vi "main.vi"(8 "error in (no error)":errorcluster) -> (0 "error out":errorcluster)   [LabVIEW 2015, in "lv-interface-nre.lvlib"]
uses:
  lv-interface-nre.lvlib
  private/_controls/hmi_references.ctl
  private/_controls/hmi_states.ctl
  private/_controls/event_common.ctl
  private/_controls/event_common_command.ctl
  private/_controls/event_interface.ctl
  private/_controls/event_interface_command.ctl
  private/_controls/menu_selection.ctl
panel:
  out "time_date":dbl format="%<%H:%M:%S%3u\n%m/%d/%y>T"
  in  "refresh_rate_ms":i32=1000
  out "random_number":dbl
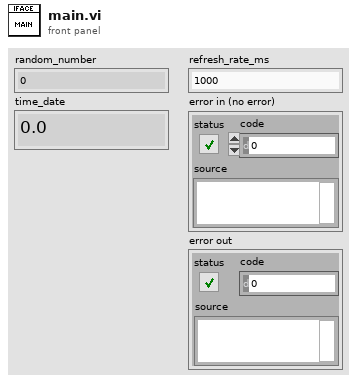
[diagram p1: front panel]
types:
  T1 = typedef "lv-interface-nre.lvlib/hmi_references.ctl" = cluster{"vi_reference":refnum<vi>}
  T2 = typedef "lv-interface-nre.lvlib/event_interface.ctl" = cluster{"command":T3, "data":variant}
  T3 = typedef "lv-interface-nre.lvlib/event_interface_command.ctl" = enum16{"<event_interface_cmd>", "defer_panel_updates", "undefer_panel_updates", "<null>"}
  T4 = typedef "lv-interface-nre.lvlib/event_common.ctl" = cluster{"command":T5, "data":variant}
  T5 = typedef "lv-interface-nre.lvlib/event_common_command.ctl" = enum16{"<event_common_cmd>", "die", "<null>"}
  T6 = typedef "lv-interface-nre.lvlib/hmi_states.ctl" = enum16{"<hmi_states>", "initialize", "checkui", "shutdown", "<null>"}
  T7 = typedef "lv-interface-nre.lvlib/menu_selection.ctl" = enum16{"<menu>", "file_exit", "help_about", "<null>"}
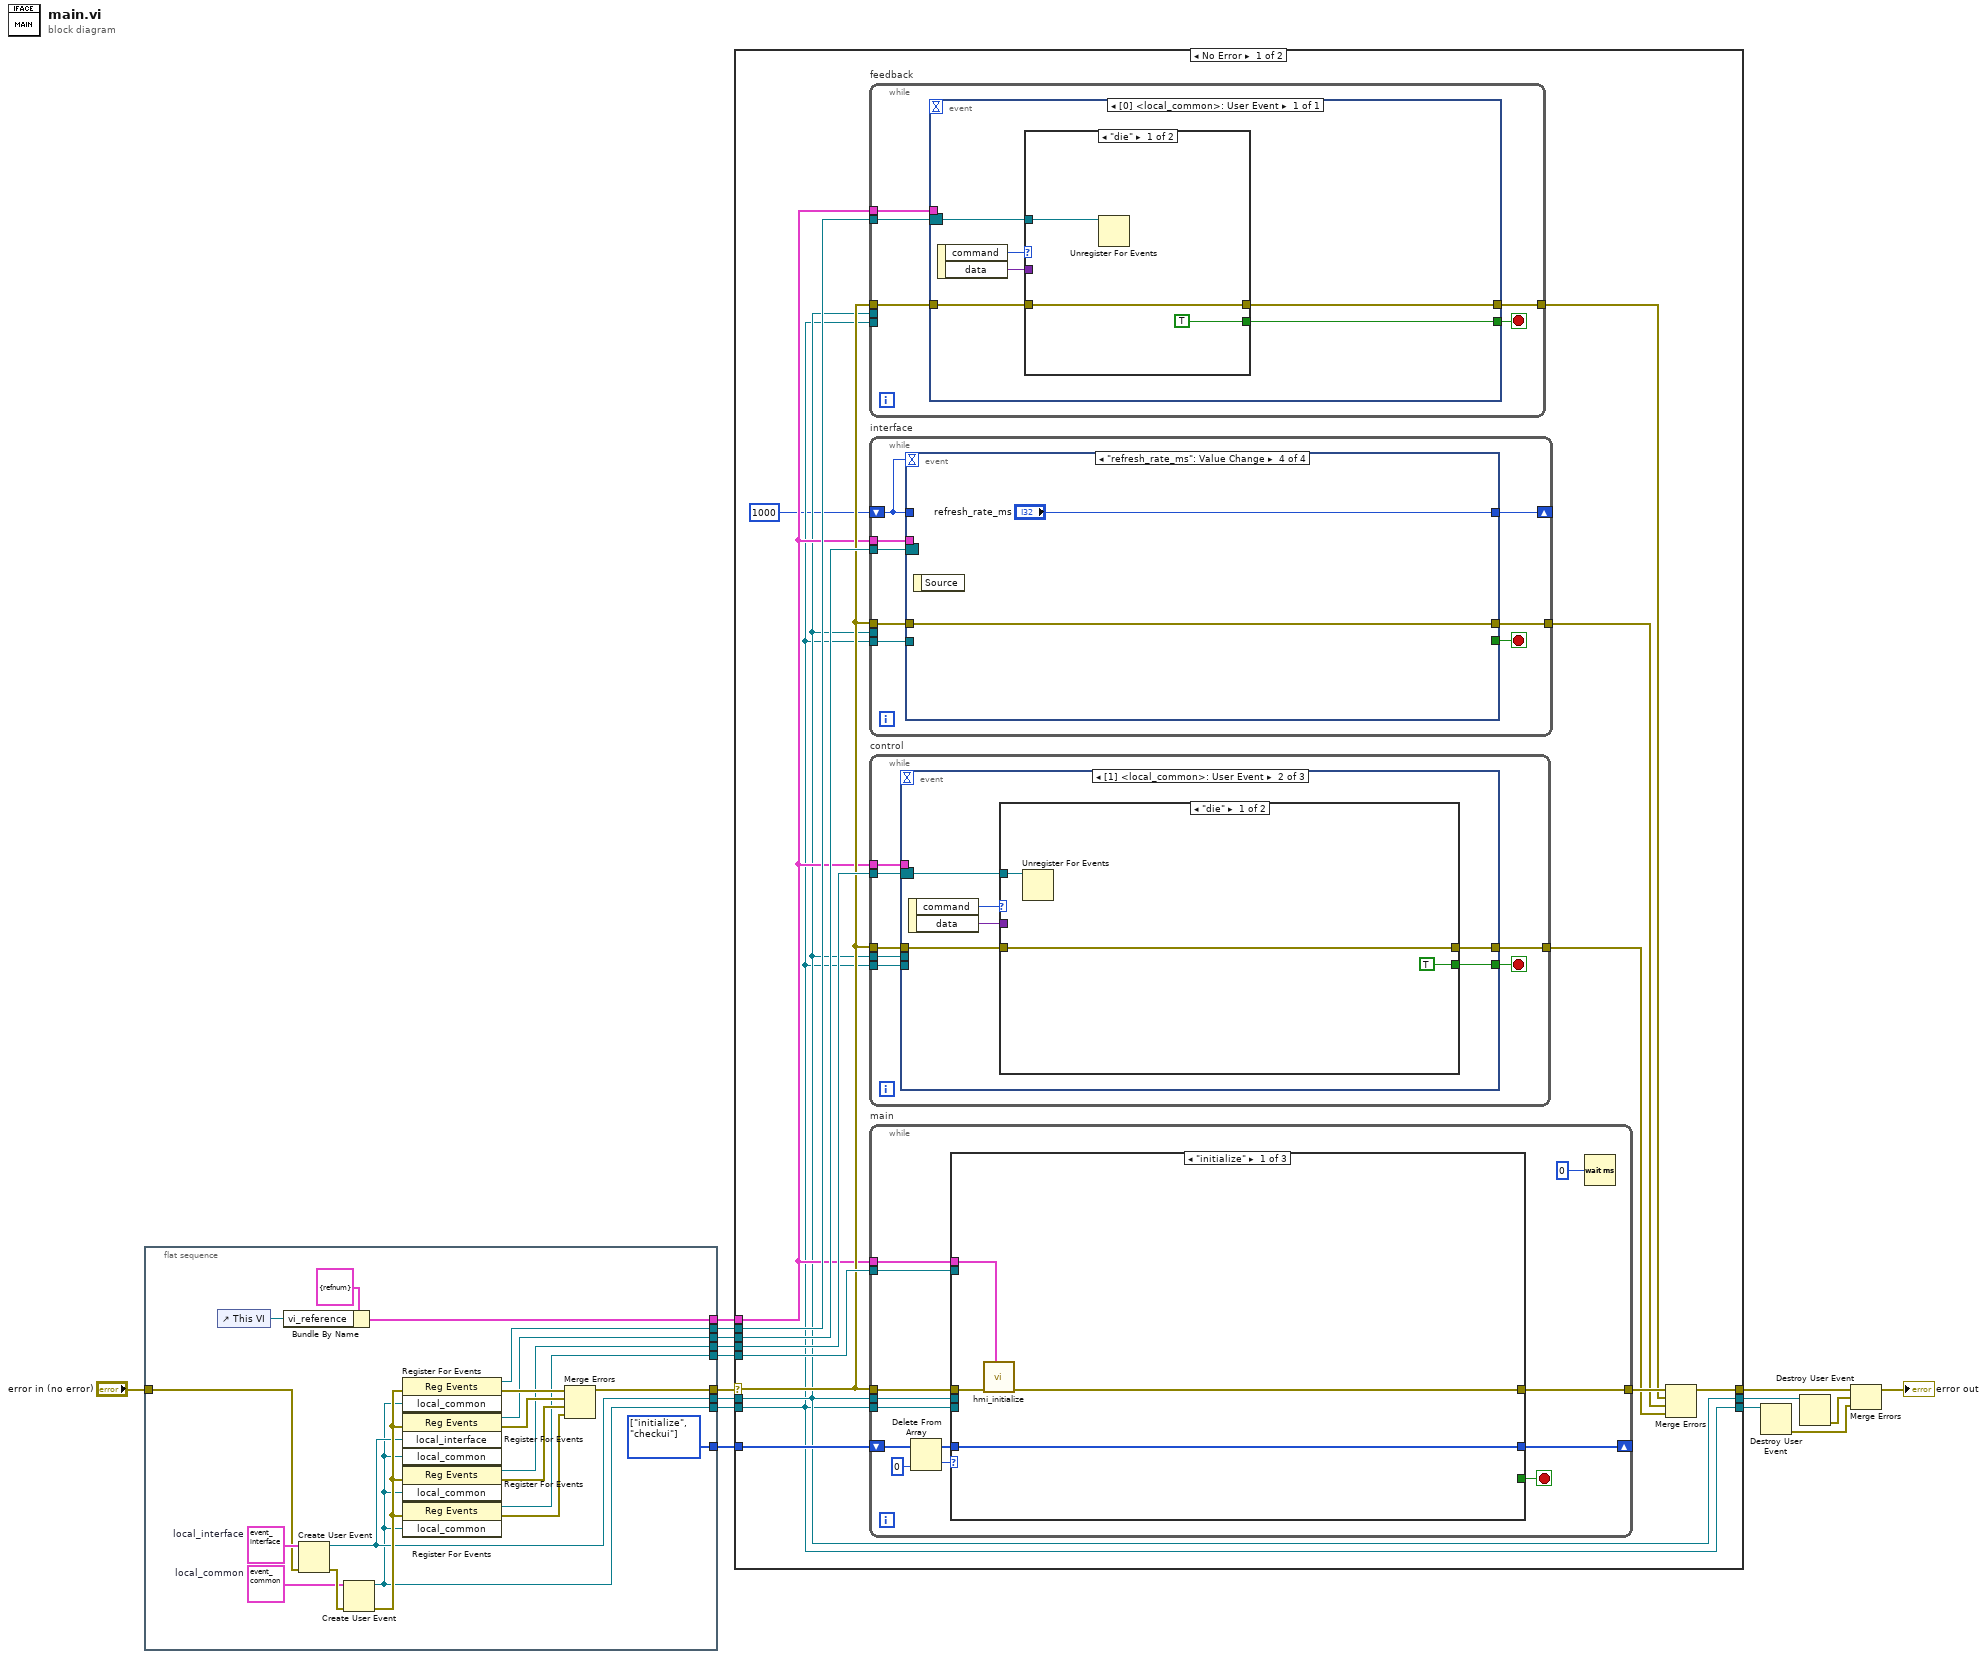
[diagram p0: block diagram]
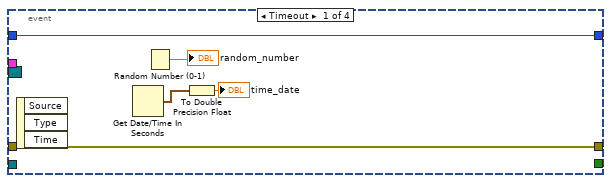
[diagram p3: hidden frame]
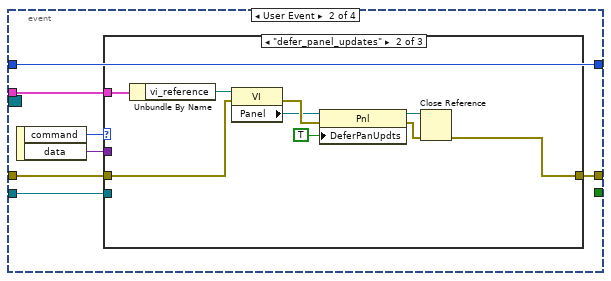
[diagram p4: hidden frame]
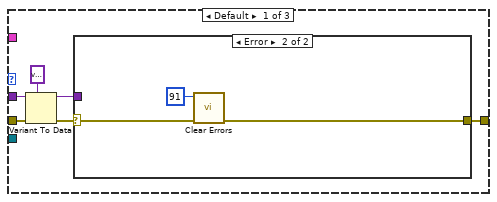
[diagram p5: hidden frame]
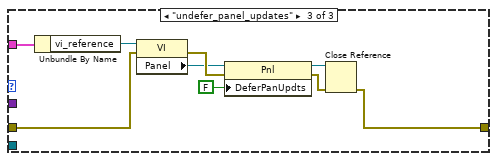
[diagram p7: hidden frame]
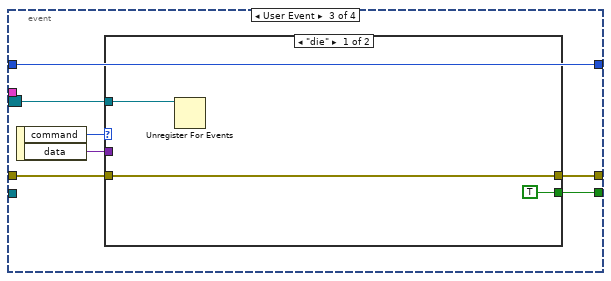
[diagram p8: hidden frame]
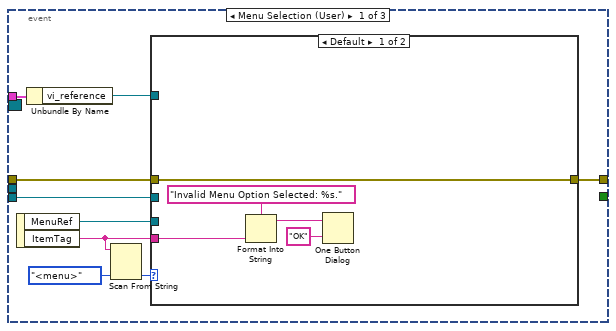
[diagram p10: hidden frame]
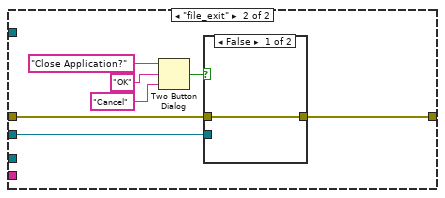
[diagram p11: hidden frame]
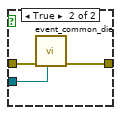
[diagram p12: hidden frame]
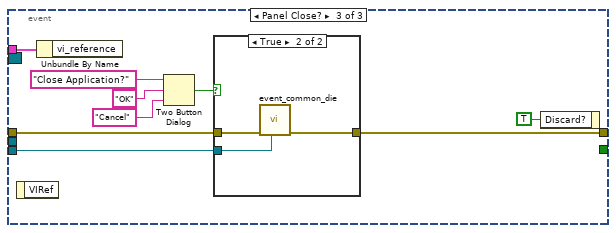
[diagram p14: hidden frame]
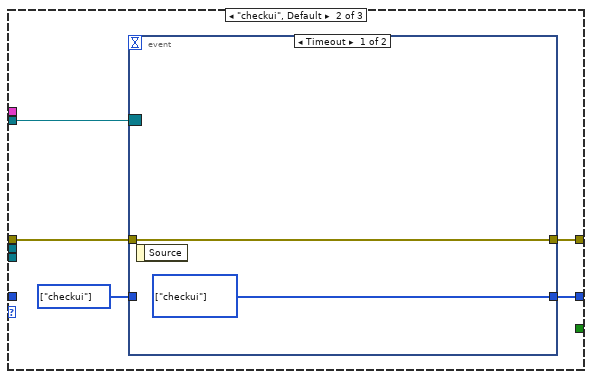
[diagram p16: hidden frame]
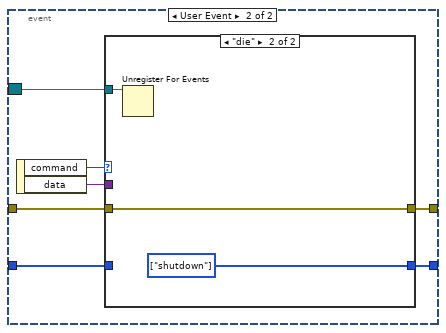
[diagram p17: hidden frame]
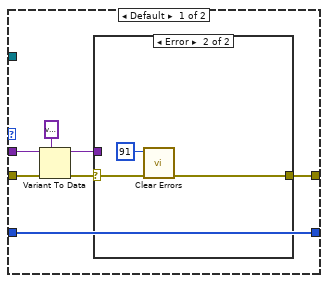
[diagram p18: hidden frame]
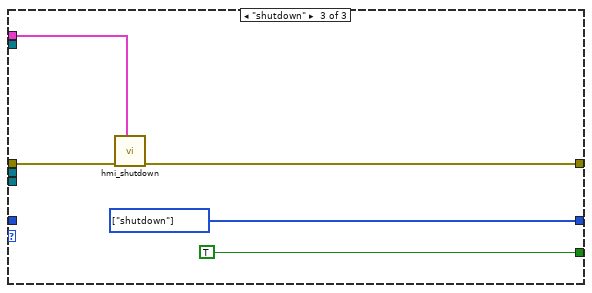
[diagram p20: hidden frame]
diagram:
  n1 = flat-sequence {
    tunnel: [w28] -> w16
    tunnel: [w27] -> w15
    tunnel: [w31] -> w14
    tunnel: "error in (no error)" -> [w17]
    tunnel: [w26] -> w12
    tunnel: [w25] -> w11
    tunnel: [w23] -> w10
    tunnel: [w19] -> w8
    tunnel: [w20] -> w9
    tunnel: [w18] -> w2
    frame #0 {
      w21 = T2 {"command"=enum."<event_interface_cmd>", "data"=variant}  # local_interface
      w22 = T4 {"command"=enum."<event_common_cmd>", "data"=variant}  # local_common
      w31 = T6[] [enum."initialize", enum."checkui"] items=["<hmi_states>", "initialize", "checkui", "shutdown", "<null>"]
      n2 = control-ref of="This VI"() -> (w24:refnum<vi>)
      n3 = Bundle By Name(cluster=T1 {"vi_reference"=refnum}, "vi_reference"=w24) -> (w23:T1)
      n4 = Create User Event(user event datatype=w21, error in=w17) -> (user event=w20:refnum<user-event>, error out=w35:errorcluster)
      n5 = Create User Event(user event datatype=w22, error in=w35) -> (user event=w19:refnum<user-event>, error out=w34:errorcluster)
      n6 = register-events(error in=w34, w19) -> (reference out=w18:refnum<event-registration>, error out=w36:errorcluster)  [unwired: 1 in]
      n7 = register-events(error in=w34, w20, w19) -> (reference out=w25:refnum<event-registration>, error out=w33:errorcluster)  [unwired: 1 in]
      n8 = register-events(error in=w34, w19) -> (reference out=w27:refnum<event-registration>, error out=w30:errorcluster)  [unwired: 1 in]
      n9 = register-events(error in=w34, w19) -> (reference out=w26:refnum<event-registration>, error out=w29:errorcluster)  [unwired: 1 in]
      n10 = Merge Errors(w36, w33, w30, w29) -> (w28:errorcluster)
    }
  }
  n11 = case shown="No Error" w16 {
    selector: w16 -> [w42 w239]
    tunnel: w15 -> [w45 w235]
    tunnel: w14 -> [w47 _]
    tunnel: [w43 w239] -> w5
    tunnel: w12 -> [w46 w234]
    tunnel: w11 -> [w44 w236]
    tunnel: w10 -> [w41 _]
    tunnel: w9 -> [w40 w238]
    tunnel: w8 -> [w39 w237]
    tunnel: [w40 w238] -> w6
    tunnel: [w39 w237] -> w7
    tunnel: w2 -> [w51 w233]
    frame No Error {
      n12 = while "feedback" {
        tunnel: [w56] -> w38
        tunnel: w42 -> [w55]
        tunnel: w51 -> [w54]
        tunnel: w41 -> [w53]
        tunnel: w40 -> [_]
        tunnel: w39 -> [_]
        stop <- w52 stop-if-true
        n13 = event shown="[0] <local_common>: User Event" {
          selector: w54 -> [w62]
          dyn-events: _ -> [_]
          timeout: _ -> [_]
          tunnel: [w59] -> w56
          tunnel: w55 -> [w60]
          tunnel: w53 -> [_]
          tunnel: [w58] -> w52
          event User Event {
            n14 = event-data() -> ("command"=w61:T5, "data"=w57:variant)  [unwired: 1 in]
            n15 = case shown="\"die\"" w61 {
              tunnel: w60 -> [w64 w66]
              tunnel: [w64 w66] -> w59
              tunnel: [TRUE _] -> w58
              tunnel: w62 -> [w63 _]
              tunnel: w57 -> [_ _]
              frame "die" {
                n16 = Unregister For Events(event registration refnum=w63) -> ()  [unwired: 1 in, 1 out]
              }
              frame Default {
              }
            }
          }
        }
      }
      n17 = while "interface" {
        tunnel: w42 -> [w74]
        tunnel: [w72] -> w48
        tunnel: w44 -> [w71]
        tunnel: w40 -> [_]
        tunnel: w39 -> [w70]
        tunnel: w41 -> [w69]
        shift-right: [w67] -> _
        shift-left: 1000 ("refresh_rate_ms") -> [w68]
        stop <- w73 stop-if-true
        n18 = event shown="[3] \"refresh_rate_ms\": Value Change" {
          selector: w71 -> [_ _ w117 _]
          dyn-events: _ -> [_ _ _ _]
          timeout: w68 -> [_ _ _ _]
          tunnel: w74 -> [w77 w84 w120 w126]
          tunnel: [w77 w83 w119 w126] -> w72
          tunnel: [_ _ w118 _] -> w73
          tunnel: w70 -> [_ w82 _ _]
          tunnel: w69 -> [_ w81 _ _]
          tunnel: w68 -> [w79 w80 w115 _]
          tunnel: [w79 w80 w115 "refresh_rate_ms"] -> w67
          event Timeout {
            n19 = event-data() -> ()  [unwired: 1 in, 3 out]
            n20 = Get Date/Time In Seconds() -> (seconds since 1Jan1904=w76:timestamp)
            n21 = Random Number (0-1)() -> (number: 0 to 1=→"random_number":dbl)
            n22 = To Double Precision Float(number=w76) -> (double precision float=→"time_date":dbl)
          }
          event User Event {
            n23 = event-data() -> ("command"=w86:T3, "data"=w85:variant)  [unwired: 1 in]
            n24 = case shown="\"defer_panel_updates\"" w86 {
              tunnel: w84 -> [w91 w100 w109]
              tunnel: [w87 w99 w106] -> w83
              tunnel: w85 -> [w92 _ _]
              tunnel: w82 -> [_ _ _]
              tunnel: w81 -> [_ w98 w108]
              frame Default {
                n25 = Variant To Data(error in=w91, type=variant, Variant=w92) -> (data=w88:variant, error out=w90:errorcluster)
                n26 = case shown="Error" w90 {
                  selector: w90 -> [w93 w96]
                  tunnel: w88 -> [_ _]
                  tunnel: [w93 w95] -> w87
                  frame No Error {
                  }
                  frame Error {
                    n27 = call <vilib>:"Clear Errors.vi"("error in (no error)"=w96, "specific error code to clear (0: all)"=91) -> ("error out"=w95:errorcluster)  [unwired: 4 in, 1 out]
                  }
                }
              }
              frame "defer_panel_updates" {
                n28 = Unbundle By Name(w98) -> ("vi_reference"=w97:refnum<vi>)
                n29 = property class="VI"(reference=w97, error in=w100) -> (error out=w105:errorcluster, "Panel"=w101:refnum<vi>)  [unwired: 1 out]
                n30 = property class="Pnl"(reference=w101, error in=w105, "DeferPanUpdts"=TRUE ("Defer Panel Updates")) -> (reference out=w103:refnum<vi>, error out=w102:errorcluster)
                n31 = Close Reference(reference=w103, error in (no error)=w102) -> (error out=w99:errorcluster)
              }
              frame "undefer_panel_updates" {
                n32 = Unbundle By Name(w108) -> ("vi_reference"=w107:refnum<vi>)
                n33 = property class="VI"(reference=w107, error in=w109) -> (error out=w114:errorcluster, "Panel"=w110:refnum<vi>)  [unwired: 1 out]
                n34 = property class="Pnl"(reference=w110, error in=w114, "DeferPanUpdts"=FALSE ("Defer Panel Updates")) -> (reference out=w112:refnum<vi>, error out=w111:errorcluster)
                n35 = Close Reference(reference=w112, error in (no error)=w111) -> (error out=w106:errorcluster)
              }
            }
          }
          event User Event {
            n36 = event-data() -> ("command"=w121:T5, "data"=w116:variant)  [unwired: 1 in]
            n37 = case shown="\"die\"" w121 {
              tunnel: w120 -> [w123 w125]
              tunnel: [w123 w125] -> w119
              tunnel: [TRUE _] -> w118
              tunnel: w117 -> [w122 _]
              tunnel: w116 -> [_ _]
              frame "die" {
                n38 = Unregister For Events(event registration refnum=w122) -> ()  [unwired: 1 in, 1 out]
              }
              frame Default {
              }
            }
          }
          event "refresh_rate_ms": Value Change {
            n39 = event-data() -> ()  [unwired: 1 in, 1 out]
          }
        }
      }
      n40 = while "control" {
        tunnel: w42 -> [w134]
        tunnel: [w132] -> w49
        tunnel: w45 -> [w131]
        tunnel: w40 -> [w129]
        tunnel: w39 -> [w128]
        tunnel: w41 -> [w130]
        stop <- w133 stop-if-true
        n41 = event shown="[1] <local_common>: User Event" {
          selector: w131 -> [_ w160 _]
          dyn-events: _ -> [_ _ _]
          timeout: _ -> [_ _ _]
          tunnel: w134 -> [w140 w164 w170]
          tunnel: [w138 w163 w177] -> w132
          tunnel: [_ w162 _] -> w133
          tunnel: w130 -> [w137 _ w176]
          tunnel: w129 -> [_ _ _]
          tunnel: w128 -> [w135 _ w175]
          event Menu Selection (User) {
            n42 = event-data() -> ("MenuRef"=w141:refnum<k9>, "ItemTag"=w139:string)  [unwired: 1 in]
            n43 = Unbundle By Name(w137) -> ("vi_reference"=w136:refnum<vi>)
            n44 = Scan From String(input string=w139, default 1=menu_selection."<menu>" ("menu_selection")) -> (output 1=w142:T7)  [unwired: 3 in, 3 out]
            n45 = case shown="Default" w142 {
              tunnel: w141 -> [_ _]
              tunnel: w140 -> [w144 w149]
              tunnel: w139 -> [w148 _]
              tunnel: [w144 w155] -> w138
              tunnel: w136 -> [_ _]
              tunnel: w135 -> [_ w154]
              frame Default {
                n46 = Format Into String(format string="Invalid Menu Option Selected: %s.", w148) -> (resulting string=w146:string)  [unwired: 2 in, 1 out]
                n47 = One Button Dialog(message=w146, button name ("OK")="OK" ("boolean_text_1")) -> ()  [unwired: 1 out]
              }
              frame "file_exit" {
                n48 = Two Button Dialog(message="Close Application?" ("dialog_text"), 1:"Cancel" ("boolean_text_1"), 2:"OK" ("boolean_text_1")) -> (T button?=w150:bool)
                n49 = case shown="False" w150 {
                  tunnel: w149 -> [w156 w159]
                  tunnel: [w156 w158] -> w155
                  tunnel: w154 -> [_ w157]
                  frame False {
                  }
                  frame True {
                    n50 = call "event_common_die.vi"("local_common"=w157, "error in (no error)"=w159) -> ("error out"=w158:errorcluster)  [unwired: 9 in]
                  }
                }
              }
            }
          }
          event User Event {
            n51 = event-data() -> ("command"=w165:T5, "data"=w161:variant)  [unwired: 1 in]
            n52 = case shown="\"die\"" w165 {
              tunnel: w164 -> [w166 w169]
              tunnel: [w166 w169] -> w163
              tunnel: [TRUE _] -> w162
              tunnel: w161 -> [_ _]
              tunnel: w160 -> [w167 _]
              frame "die" {
                n53 = Unregister For Events(event registration refnum=w167) -> ()  [unwired: 1 in, 1 out]
              }
              frame Default {
              }
            }
          }
          event Panel Close? {
            n54 = event-data() -> ()  [unwired: 1 in, 1 out]
            n55 = Unbundle By Name(w176) -> ()  [unwired: 1 out]
            n56 = Two Button Dialog(message="Close Application?" ("dialog_text"), 1:"Cancel" ("boolean_text_1"), 2:"OK" ("boolean_text_1")) -> (T button?=w171:bool)
            n57 = case shown="True" w171 {
              tunnel: w170 -> [w179 w182]
              tunnel: [w179 w181] -> w177
              tunnel: w175 -> [_ w180]
              frame False {
              }
              frame True {
                n58 = call "event_common_die.vi"("local_common"=w180, "error in (no error)"=w182) -> ("error out"=w181:errorcluster)  [unwired: 9 in]
              }
            }
            n59 = event-data("Discard?"=TRUE) -> ()  [unwired: 1 in, 1 out]
          }
        }
      }
      n60 = while "main" {
        shift-right: [w187] -> _
        shift-left: w47 -> [w194]
        tunnel: w46 -> [w188]
        tunnel: w42 -> [w190]
        tunnel: [w186] -> w50
        tunnel: w41 -> [w185]
        tunnel: w39 -> [w184]
        tunnel: w40 -> [w183]
        stop <- w189 stop-if-true
        n61 = Delete From Array(array=w194, index=0) -> (deleted portion=w192:T6, array with subset deleted=w191:T6[])  [unwired: 1 in]
        n62 = case shown="\"initialize\"" w192 {
          tunnel: w191 -> [w199 _ _]
          tunnel: w190 -> [w198 w204 w231]
          tunnel: [_ _ TRUE] -> w189
          tunnel: [w196 w203 w230] -> w186
          tunnel: [w199 w202 w229] -> w187
          tunnel: w188 -> [_ w200 _]
          tunnel: w185 -> [w197 _ w228]
          tunnel: w184 -> [_ _ _]
          tunnel: w183 -> [_ _ _]
          frame "initialize" {
            n63 = call "hmi_initialize.vi"("hmi_references"=w197, "error in (no error)"=w198) -> ("error out"=w196:errorcluster)  [unwired: 9 in]
          }
          frame "checkui", Default {
            w201 = T6[] [enum."checkui"] items=["<hmi_states>", "initialize", "checkui", "shutdown", "<null>"]
            n64 = event shown="[0] Timeout" {
              selector: w200 -> [_ w207]
              dyn-events: _ -> [_ _]
              timeout: _ -> [_ _]
              tunnel: w204 -> [w206 w211]
              tunnel: [w206 w208] -> w203
              tunnel: [w205 w209] -> w202
              tunnel: w201 -> [_ w210]
              event Timeout {
                w205 = T6[] [enum."checkui"] items=["<hmi_states>", "initialize", "checkui", "shutdown", "<null>"]
                n65 = event-data() -> ()  [unwired: 1 in, 1 out]
              }
              event User Event {
                n66 = event-data() -> ("command"=w213:T5, "data"=w212:variant)  [unwired: 1 in]
                n67 = case shown="\"die\"" w213 {
                  tunnel: [w220 w227] -> w209
                  tunnel: w210 -> [w220 _]
                  tunnel: w211 -> [w218 w226]
                  tunnel: [w214 w226] -> w208
                  tunnel: w212 -> [w219 _]
                  tunnel: w207 -> [_ w225]
                  frame Default {
                    n68 = Variant To Data(error in=w218, type=variant, Variant=w219) -> (data=w215:variant, error out=w217:errorcluster)
                    n69 = case shown="Error" w217 {
                      selector: w217 -> [w221 w224]
                      tunnel: w215 -> [_ _]
                      tunnel: [w221 w223] -> w214
                      frame No Error {
                      }
                      frame Error {
                        n70 = call <vilib>:"Clear Errors.vi"("error in (no error)"=w224, "specific error code to clear (0: all)"=91) -> ("error out"=w223:errorcluster)  [unwired: 4 in, 1 out]
                      }
                    }
                  }
                  frame "die" {
                    w227 = T6[] [enum."shutdown"] items=["<hmi_states>", "initialize", "checkui", "shutdown", "<null>"]
                    n71 = Unregister For Events(event registration refnum=w225) -> ()  [unwired: 1 in, 1 out]
                  }
                }
              }
            }
          }
          frame "shutdown" {
            w229 = T6[] [enum."shutdown"] items=["<hmi_states>", "initialize", "checkui", "shutdown", "<null>"]
            n72 = call "hmi_shutdown.vi"("hmi_references"=w228, "error in (no error)"=w231) -> ("error out"=w230:errorcluster)  [unwired: 9 in]
          }
        }
        n73 = Wait (ms)(milliseconds to wait=u32 0) -> ()  [unwired: 1 out]
      }
      n74 = Merge Errors(w50, w38, w48, w49) -> (w43:errorcluster)
    }
    frame Error {
      n75 = Unregister For Events(event registration refnum=w234) -> ()  [unwired: 1 in, 1 out]
      n76 = Unregister For Events(event registration refnum=w235) -> ()  [unwired: 1 in, 1 out]
      n77 = Unregister For Events(event registration refnum=w236) -> ()  [unwired: 1 in, 1 out]
      n78 = Unregister For Events(event registration refnum=w233) -> ()  [unwired: 1 in, 1 out]
    }
  }
  n79 = Destroy User Event(user event=w7) -> (error out=w3:errorcluster)  [unwired: 1 in]
  n80 = Destroy User Event(user event=w6) -> (error out=w4:errorcluster)  [unwired: 1 in]
  n81 = Merge Errors(w5, w4, w3) -> (→"error out":errorcluster)
